vi "svx_DAQ_ConfigureTiming.vi"(0 "Task In":refnum<k21>, 5 "Display State In":T2={"Channel Info Array"=[], "Timing Mode"=enum."Time", "Timing Control 1"=25600.0, "Timing Control 2"=2560.0, "Timing Control 3"=16, "Timing Indicator 1"=0.1, "Reference Visible?"=FALSE, "Reference Type"=enum."<none>", "Tachometer Channel"="", "Tach Pulses Per Rev"=1, "Tach Direction"=enum."CW", "Tach Slope"=enum."Rising", "Tach Threshold"=0.0, "Trigger Channel"="", "Trigger Level"=20.0, "Pretrigger Samples"=1, "Trigger Slope"=enum."Falling", "Trigger Hysteresis"=0.0, "Logging Visible?"=FALSE, "Enable Logging"=FALSE, "Logfile Path"=path "c:/test.tdms"} caption="State" {"Timing Control 2" format="%#_6f"; "Channel Info Array"."Max" min=0.0 format="± %^#_4g"; "Channel Info Array"."Channel Type" items=["Voltage (V)"=0, "Charge (C)"=9, "-"=99, "SPL (Pa)"=3, "Force (lbf)"=6, "Force (N)"=1, "Acceleration (g) - IEPE"=2, "Acceleration (g) - Charge"=12, "Acceleration (g) - 4 wire DC Voltage"=22, "Velocity (in/s)"=7, "Velocity (mm/s)"=8, "Prox Probe (mil)"=4, "Prox Probe (mm)"=5]}, 9 "cluster":T1, 11 "Error In (no error)":errorcluster) -> (4 "task out":refnum<k21>, 6 "Display State Out":T2={"Channel Info Array"=[], "Timing Mode"=enum."Time", "Timing Control 1"=25600.0, "Timing Control 2"=2560.0, "Timing Control 3"=16, "Timing Indicator 1"=0.1, "Reference Visible?"=FALSE, "Reference Type"=enum."<none>", "Tachometer Channel"="", "Tach Pulses Per Rev"=1, "Tach Direction"=enum."CW", "Tach Slope"=enum."Rising", "Tach Threshold"=0.0, "Trigger Channel"="", "Trigger Level"=20.0, "Pretrigger Samples"=1, "Trigger Slope"=enum."Falling", "Trigger Hysteresis"=0.0, "Logging Visible?"=FALSE, "Enable Logging"=FALSE, "Logfile Path"=path "c:/test.tdms"} caption="State" {"Timing Control 2" format="%#_6f"; "Channel Info Array"."Max" min=0.0 format="± %^#_4g"; "Channel Info Array"."Channel Type" items=["Voltage (V)"=0, "Charge (C)"=9, "-"=99, "SPL (Pa)"=3, "Force (lbf)"=6, "Force (N)"=1, "Acceleration (g) - IEPE"=2, "Acceleration (g) - Charge"=12, "Acceleration (g) - 4 wire DC Voltage"=22, "Velocity (in/s)"=7, "Velocity (mm/s)"=8, "Prox Probe (mil)"=4, "Prox Probe (mm)"=5]}, 10 "cluster":T1, 15 "error out":errorcluster)   [LabVIEW 2017, in "SVX NI-DAQmx AI Configuration XControl.xctl"]
uses:
  <vilib>/addons/Sound and Vibration/svt_DAQmx/Configuration XControl/SVX NI-DAQmx AI Configuration XControl.xctl
  <vilib>/addons/Sound and Vibration/svt_DAQmx/Configuration XControl/SubVIs/svx_DAQ_State.ctl
  <vilib>/addons/Sound and Vibration/svt_DAQmx/Configuration XControl/Controls/svx_DAQ_ChannelInfo.ctl
  <vilib>/addons/Sound and Vibration/svt_DAQmx/Configuration XControl/Controls/svx_DAQ_ChannelType.ctl
  <vilib>/addons/Sound and Vibration/svt_DAQmx/Configuration XControl/Controls/svx_DAQ_Coupling.ctl
  <vilib>/addons/Sound and Vibration/svt_DAQmx/Configuration XControl/Controls/svx_DAQ_Excitation.ctl
  <vilib>/addons/Sound and Vibration/svt_DAQmx/Configuration XControl/Controls/svx_DAQ_TimingType.ctl
  <vilib>/addons/Sound and Vibration/svt_DAQmx/Configuration XControl/Controls/svx_DAQ_ReferenceType.ctl
  <vilib>/addons/Sound and Vibration/svt_DAQmx/Configuration XControl/Controls/svx_DAQ_RotationDirection.ctl
  <vilib>/addons/Sound and Vibration/svt_DAQmx/Configuration XControl/Controls/svx_DAQ_Tach_Slope.ctl
  <vilib>/addons/Sound and Vibration/svt_DAQmx/Configuration XControl/Controls/svx_DAQ_Trigger_Slope.ctl
  <vilib>/addons/Sound and Vibration/svt_DAQmx/Configuration XControl/Controls/svx_DAQ_ControlRefs.ctl
  <resource>/objmgr/daqmx.rc
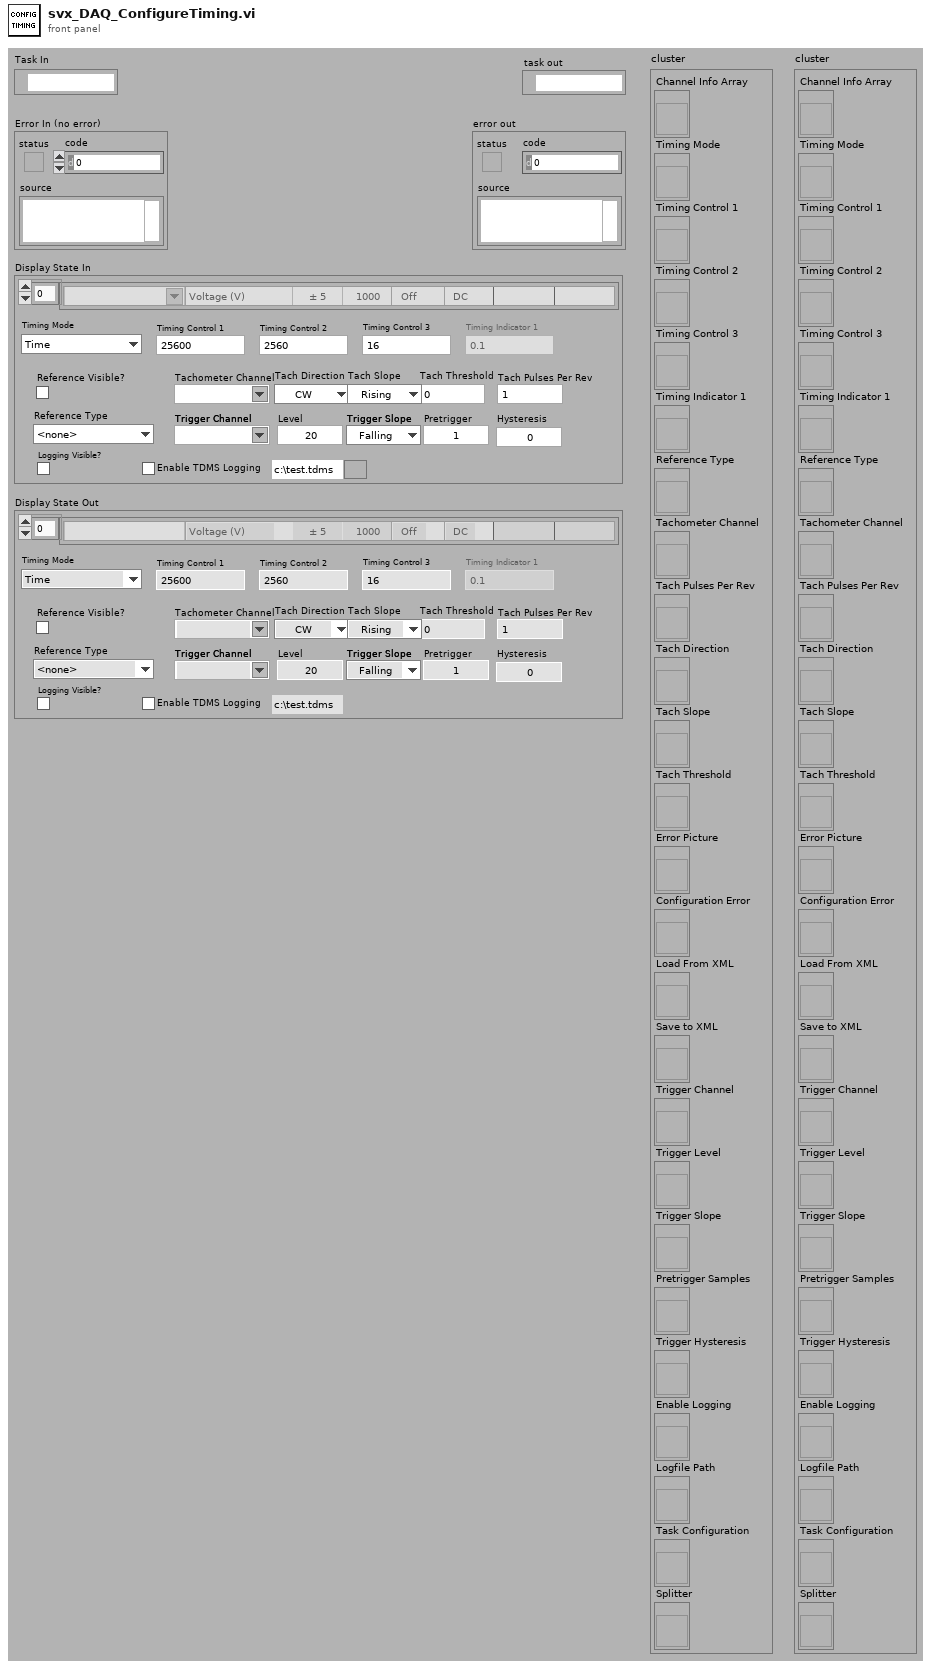
[diagram p1: front panel]
types:
  T1 = typedef "SVX NI-DAQmx AI Configuration XControl.xctl/svx_DAQ_ControlRefs.ctl" = cluster{"Channel Info Array":refnum<vi>, "Timing Mode":refnum<vi>, "Timing Control 1":refnum<vi>, "Timing Control 2":refnum<vi>, "Timing Control 3":refnum<vi>, "Timing Indicator 1":refnum<vi>, "Reference Type":refnum<vi>, "Tachometer Channel":refnum<vi>, "Tach Pulses Per Rev":refnum<vi>, "Tach Direction":refnum<vi>, "Tach Slope":refnum<vi>, "Tach Threshold":refnum<vi>, "Error Picture":refnum<vi>, "Configuration Error":refnum<vi>, "Load From XML":refnum<vi>, "Save to XML":refnum<vi>, "Trigger Channel":refnum<vi>, "Trigger Level":refnum<vi>, "Trigger Slope":refnum<vi>, "Pretrigger Samples":refnum<vi>, "Trigger Hysteresis":refnum<vi>, "Enable Logging":refnum<vi>, "Logfile Path":refnum<vi>, "Task Configuration":refnum<vi>, "Splitter":refnum<vi>}
  T2 = typedef "SVX NI-DAQmx AI Configuration XControl.xctl/svx_DAQ_State.ctl" = cluster{"Channel Info Array":T3[], "Timing Mode":T7, "Timing Control 1":dbl, "Timing Control 2":dbl, "Timing Control 3":i32, "Timing Indicator 1":dbl, "Reference Visible?":bool, "Reference Type":T8, "Tachometer Channel":string, "Tach Pulses Per Rev":i32, "Tach Direction":T9, "Tach Slope":T10, "Tach Threshold":dbl, "Trigger Channel":string, "Trigger Level":dbl, "Pretrigger Samples":i32, "Trigger Slope":T11, "Trigger Hysteresis":dbl, "Logging Visible?":bool, "Enable Logging":bool, "Logfile Path":path}
  T3 = typedef "SVX NI-DAQmx AI Configuration XControl.xctl/svx_DAQ_ChannelInfo.ctl" = cluster{"Initialized?":bool, "DAQmx Channel":tag, "Channel Type":T4, "Max":dbl, "Sensitivity":dbl, "Excitation":bool, "Coupling":T5, "Location":string, "Orientation":string, "excitation":T6}
  T4 = typedef "SVX NI-DAQmx AI Configuration XControl.xctl/svx_DAQ_ChannelType.ctl" = u16
  T5 = typedef "SVX NI-DAQmx AI Configuration XControl.xctl/svx_DAQ_Coupling.ctl" = enum16{"AC", "DC"}
  T6 = typedef "svx_DAQ_Excitation.ctl" = enum16{"Off", "Min", "Max"}
  T7 = typedef "SVX NI-DAQmx AI Configuration XControl.xctl/svx_DAQ_TimingType.ctl" = enum16{"Time", "Frequency", "Order"}
  T8 = typedef "SVX NI-DAQmx AI Configuration XControl.xctl/svx_DAQ_ReferenceType.ctl" = enum16{"<none>", "Analog Tachometer", "Analog SW Trigger"}
  T9 = typedef "SVX NI-DAQmx AI Configuration XControl.xctl/svx_DAQ_RotationDirection.ctl" = enum16{"CW", "CCW"}
  T10 = typedef "SVX NI-DAQmx AI Configuration XControl.xctl/svx_DAQ_Tach_Slope.ctl" = enum16{"Rising", "Falling"}
  T11 = typedef "SVX NI-DAQmx AI Configuration XControl.xctl/svx_DAQ_Trigger_Slope.ctl" = enum16{"Falling", "Rising"}
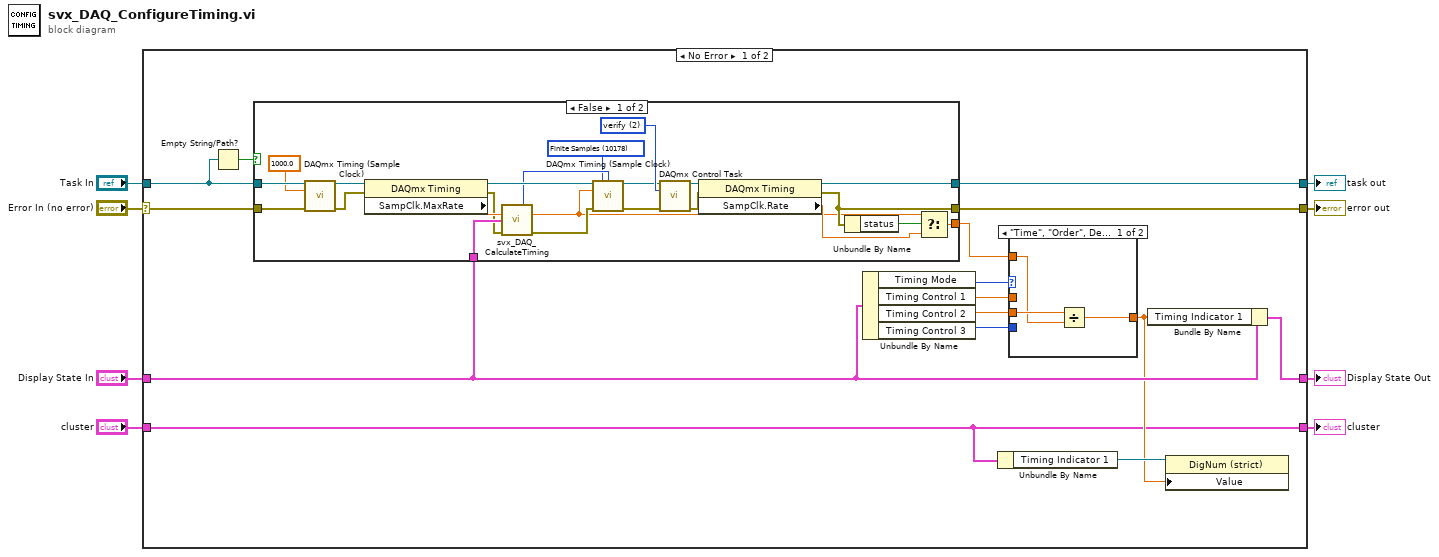
[diagram p0: block diagram]
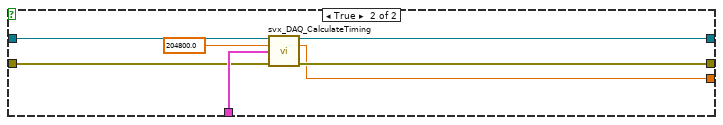
[diagram p2: hidden frame]
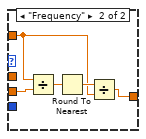
[diagram p3: hidden frame]
diagram:
  n1 = case shown="No Error" "Error In (no error)" {
    selector: "Error In (no error)" -> [w14 w64]
    tunnel: [w23 w62] -> w8
    tunnel: "Display State In" -> [w22 w62]
    tunnel: [w21 w64] -> w6
    tunnel: [w20 w63] -> w5
    tunnel: "Task In" -> [w9 w63]
    tunnel: "cluster" -> [w11 w61]
    tunnel: [w11 w61] -> w2
    frame No Error {
      n2 = Empty String/Path?(string/path=w9) -> (empty?=w10:bool)
      n3 = case shown="False" w10 {
        tunnel: w22 -> [w46 w52]
        tunnel: [w45 w50] -> w21
        tunnel: [w44 w47] -> w20
        tunnel: w9 -> [w35 w47]
        tunnel: [w42 w48] -> w19
        tunnel: w14 -> [w33 w51]
        frame False {
          w36 = 2 items=["verify"=2, "reserve"=4, "commit"=3, "unreserve"=5, "abort"=6] ("action")
          w24 = 10178 items=["Finite Samples"=10178, "Continuous Samples"=10123, "Hardware Timed Single Point"=12522] ("sample mode")
          n4 = call <vilib>:"DAQmx Timing (Sample Clock).vi"("task/channels in"=w35, "rate"=1000.0, "error in"=w33) -> ("task out"=w32:refnum<k21>, "error out"=w31:errorcluster)  [unwired: 11 in]
          n5 = property class="DAQmx Timing"(reference=w32, error in=w31) -> (reference out=w30:refnum<k21>, error out=w37:errorcluster, "SampClk.MaxRate"=w38:dbl)
          n6 = call <vilib>:"svx_DAQ_CalculateTiming.vi"("SampClk.MaxRate"=w38, "Display State In"=w46, "error in (no error)"=w37) -> ("Samples Per Channel"=w29:i32, "Sample Rate"=w27:dbl, "error out"=w28:errorcluster)  [unwired: 10 in]
          n7 = call <vilib>:"DAQmx Timing (Sample Clock).vi"("task/channels in"=w30, "sample mode"=w24, "samples per channel"=w29, "rate"=w27, "error in"=w28) -> ("task out"=w26:refnum<k21>, "error out"=w25:errorcluster)  [unwired: 9 in]
          n8 = call <vilib>:"DAQmx Control Task.vi"("task/channels in"=w26, "action"=w36, "error in"=w25) -> ("task out"=w39:refnum<k21>, "error out"=w40:errorcluster)  [unwired: 11 in]
          n9 = property class="DAQmx Timing"(reference=w39, error in=w40) -> (reference out=w44:refnum<k21>, error out=w45:errorcluster, "SampClk.Rate"=w41:dbl)
          n10 = Unbundle By Name(w45) -> ("status"=w43:bool)
          n11 = Select(t=w27, s=w43, f=w41) -> (s? t:f=w42:dbl)
        }
        frame True {
          n12 = call <vilib>:"svx_DAQ_CalculateTiming.vi"("SampClk.MaxRate"=204800.0, "Display State In"=w52, "error in (no error)"=w51) -> ("Sample Rate"=w48:dbl, "error out"=w50:errorcluster)  [unwired: 10 in, 1 out]
        }
      }
      n13 = Unbundle By Name(w22) -> ("Timing Mode"=w15:T7, "Timing Control 1"=w16:dbl, "Timing Control 2"=w17:dbl, "Timing Control 3"=w18:i32)
      n14 = Unbundle By Name(w11) -> ("Timing Indicator 1"=w13:refnum<vi>)
      n15 = case shown="\"Time\", \"Order\", Default" w15 {
        tunnel: w16 -> [_ _]
        tunnel: w17 -> [w55 w60]
        tunnel: w18 -> [_ _]
        tunnel: [w54 w56] -> w12
        tunnel: w19 -> [w53 w57]
        frame "Time", "Order", Default {
          n16 = Divide(x=w55, y=w53) -> (x/y=w54:dbl)
        }
        frame "Frequency" {
          n17 = Divide(x=w57, y=w60) -> (x/y=w59:dbl)
          n18 = Round To Nearest(number=w59) -> (nearest integer value=w58:dbl)
          n19 = Divide(x=w58, y=w57) -> (x/y=w56:dbl)
        }
      }
      n20 = Bundle By Name(cluster=w22, "Timing Indicator 1"=w12) -> (w23:T2)
      n21 = property class="DigNum (strict)"(reference=w13, "Value"=w12) -> ()  [unwired: 1 in, 2 out]
    }
    frame Error {
    }
  }
  "Display State Out" <- w8
  "error out" <- w6
  "task out" <- w5
  "cluster" <- w2
